vi "230524_ExamPractice.vi"() -> ()   [LabVIEW 2022 SP3]
uses:
  <vilib>/addons/database/Connection.llb/DB Tools Open Connec (Path).vi
  <vilib>/addons/database/_DB Variant To Data/Database Variant To Data.xnode
  <vilib>/addons/database/NI_Database_API.lvlib
panel:
  in  "stop":bool
  in  "table":string
  in  "connection information":path=path "D:/School/AIIT/4AHME/LabView/230524_ExamPractice/230524_ExamPractice.udl"
  in  "Tab Control":enum32{"Lesen", "Schreiben"}(tab)
  out "data":string[][](array[string])
  in  "Write":bool
  in  "katalognummer":string
  in  "vorname":string
  in  "nachname":string
  in  "iq":string
  in  "klasse":string
  in  "schuelernummer":string
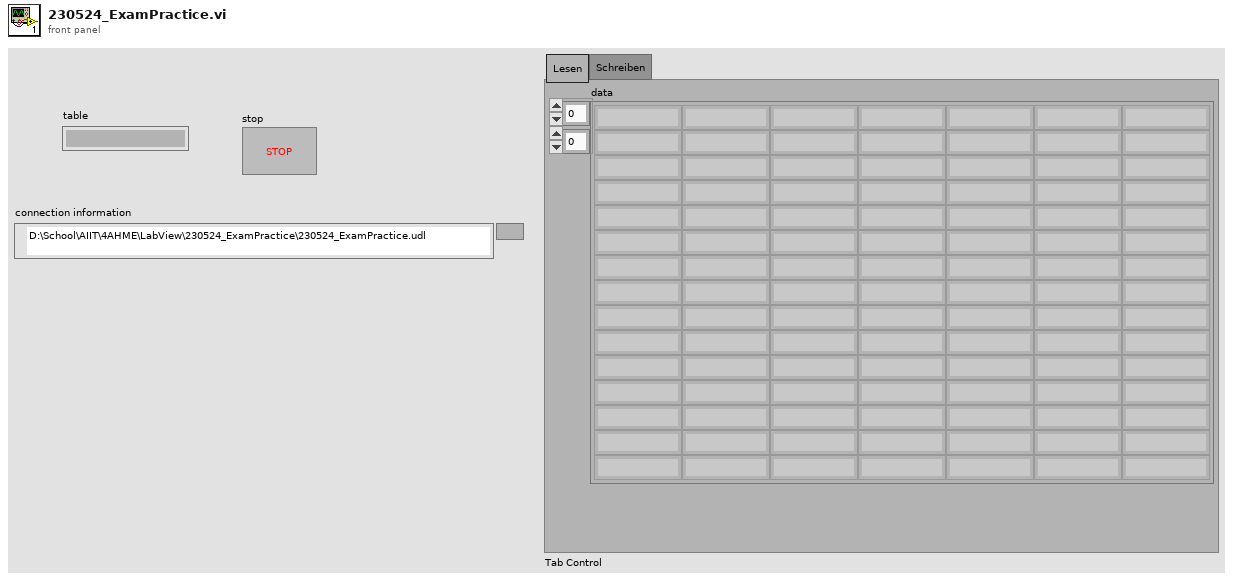
[diagram p1: front panel]
types:
  T1 = cluster{"katalognummer":string, "vorname":string, "nachname":string, "iq":string, "klasse":string, "schuelernummer":string}
  T2 = typedef "NI_Database_API.lvlib/Conn ObjectReference.ctl" = refnum<k1>
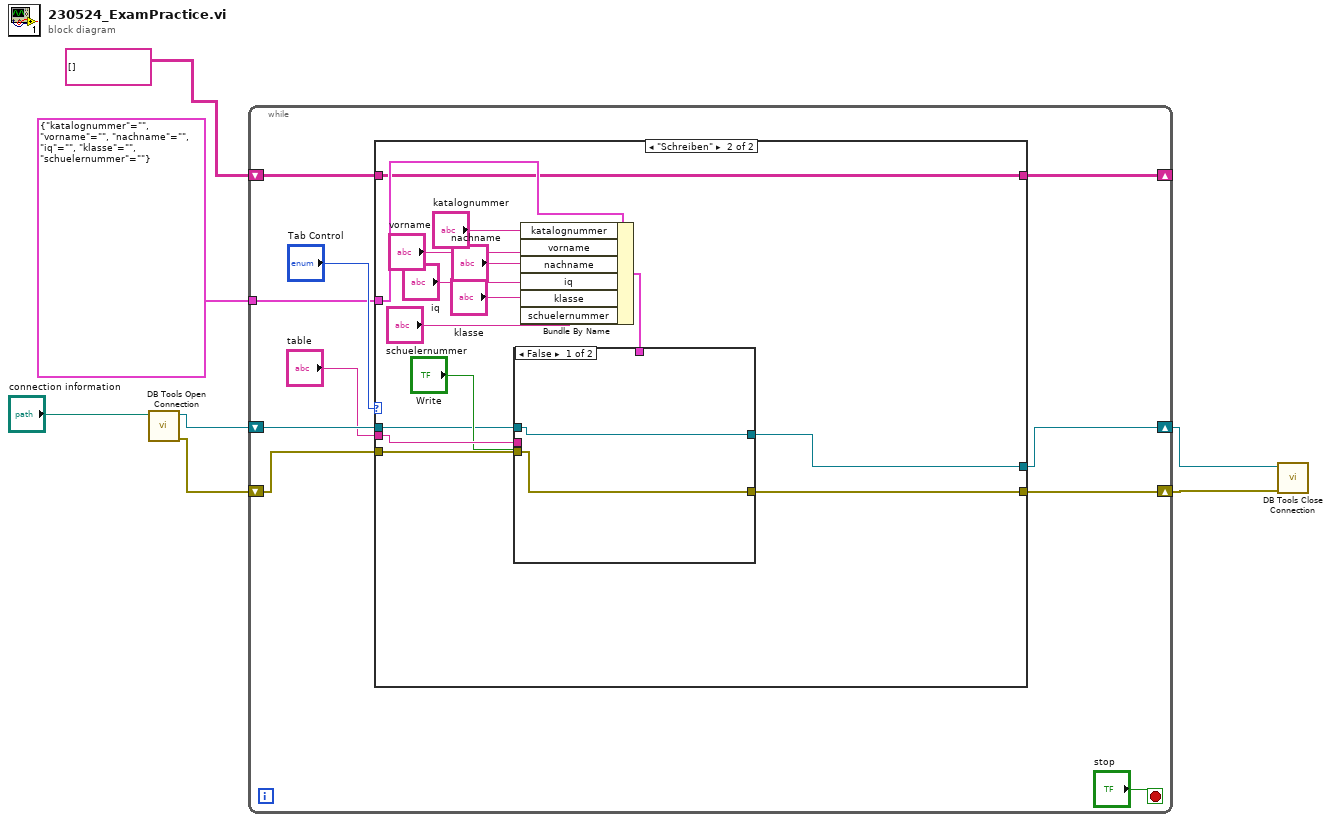
[diagram p0: block diagram]
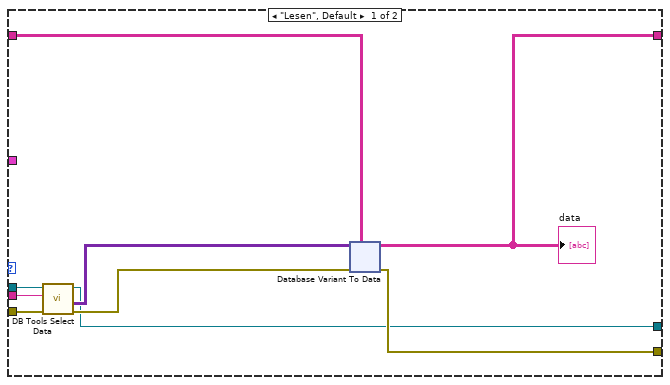
[diagram p2: hidden frame]
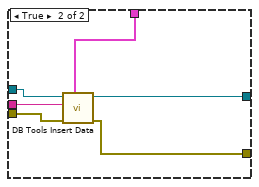
[diagram p3: hidden frame]
diagram:
  n1 = call-poly <vilib>:"DB Tools Open Connection.vi"("connection information"="connection information") -> ("error out"=w5:errorcluster, "connection reference"=w6:T2)  [unwired: 7 in]
  n2 = while {
    shift-right: [w15] -> w4
    shift-left: w5 -> [w16]
    shift-right: [w9] -> w1
    shift-left: w6 -> [w17]
    tunnel: T1 {"katalognummer"="", "vorname"="", "nachname"="", "iq"="", "klasse"="", "schuelernummer"=""} -> [w10]
    shift-right: [w8] -> _
    shift-left: string[][] [] -> [w12]
    stop <- "stop" stop-if-true
    n3 = case shown="\"Schreiben\"" "Tab Control" {
      tunnel: w17 -> [w26 w80]
      tunnel: w16 -> [w25 w82]
      tunnel: [w23 w85] -> w15
      tunnel: "table" -> [w22 w83]
      tunnel: w12 -> [w20 w71]
      tunnel: [w19 w84] -> w9
      tunnel: w10 -> [_ w79]
      tunnel: [w18 w71] -> w8
      frame "Lesen", Default {
        n4 = call <vilib>:"DB Tools Select Data.vi"("error in (no error)"=w25, "table"=w22, "connection reference"=w26) -> ("error out"=w24:errorcluster, "data"=w21:variant[][], "connection reference out"=w19:T2)  [unwired: 3 in]
        n5 = xnode "Database Variant To Data"("database variant"=w21, "error in (no error)"=w24, "type"=w20) -> ("data"=w18:string[][], "error out"=w23:errorcluster)
        "data" <- w18
      }
      frame "Schreiben" {
        n6 = Bundle By Name(cluster=w79, "katalognummer"="katalognummer", "vorname"="vorname", "nachname"="nachname", "iq"="iq", "klasse"="klasse", "schuelernummer"="schuelernummer") -> (w72:T1)
        n7 = case shown="False" "Write" {
          tunnel: [w87 w93] -> w85
          tunnel: [w86 w92] -> w84
          tunnel: w83 -> [_ w91]
          tunnel: w82 -> [w87 w90]
          tunnel: w80 -> [w86 w89]
          tunnel: w72 -> [_ w88]
          frame False {
          }
          frame True {
            n8 = call <vilib>:"DB Tools Insert Data.vi"("data"=w88, "error in (no error)"=w90, "table"=w91, "connection reference"=w89) -> ("error out"=w93:errorcluster, "connection reference out"=w92:T2)  [unwired: 6 in]
          }
        }
      }
    }
  }
  n9 = call <vilib>:"DB Tools Close Connection.vi"("error in (no error)"=w4, "connection reference"=w1) -> ()  [unwired: 5 in, 1 out]
